vi "Check Port Exposure Changed.vi"(11 "Name":string) -> ()   [LabVIEW 2023]
uses:
  Camera Set Up/Event Setup Types.ctl
  <vilib>/Rock Robotics/Network Tables/NT Read Number.vi
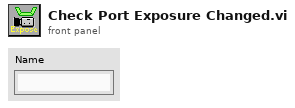
[diagram p1: front panel]
types:
  T1 = typedef "Event Setup Types.ctl" = enum16{"Save Data", "Calibrate", "Set White Balance", "Set Brightness", "Set Exposure", "Update Brightness", "Update Exposure", "Update White Balance", "Exit"}
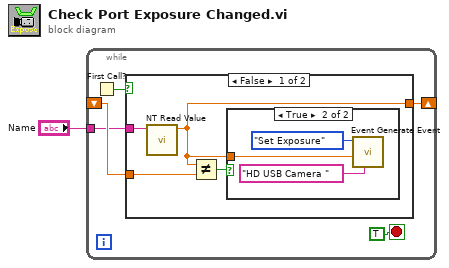
[diagram p0: block diagram]
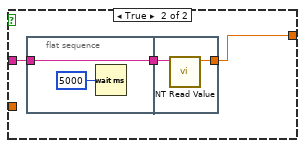
[diagram p3: hidden frame]
diagram:
  n1 = while {
    shift-right: [w6] -> _
    shift-left: _ -> [w5]
    tunnel: "Name" -> [w2]
    stop <- TRUE stop-if-true
    n2 = First Call?() -> (First Call?: T/F=w3:bool)
    n3 = case shown="False" w3 {
      tunnel: [w9 w15] -> w6
      tunnel: w5 -> [w8 _]
      tunnel: w2 -> [w7 w16]
      frame False {
        n4 = call-poly <vilib>:"NT Read Value.vi"("name"=w7) -> ("value"=w9:dbl)  [unwired: 8 in, 2 out]
        n5 = Not Equal?(x=w9, y=w8) -> (x != y?=w10:bool)
        n6 = case shown="True" w10 {
          tunnel: w9 -> [_ w11]
          frame False {
          }
          frame True {
            n7 = call "Event Generate Event.vi"("Camera Name"="HD USB Camera " ("y"), "Setpoint"=w11, "Event Type"=Event_Setup_Types."Set Exposure") -> ()  [unwired: 9 in]
          }
        }
      }
      frame True {
        n8 = flat-sequence {
          tunnel: w16 -> [w18]
          tunnel: [w18] -> w14
          tunnel: [w19] -> w15
          tunnel: w14 -> [w20]
          frame #0 {
            n9 = Wait (ms)(milliseconds to wait=u32 5000) -> ()  [unwired: 1 out]
          }
          frame #1 {
            n10 = call-poly <vilib>:"NT Read Value.vi"("name"=w20) -> ("value"=w19:dbl)  [unwired: 8 in, 2 out]
          }
        }
      }
    }
  }
